vi "Get Area Temperature.vi"(8 "error in (no error)":errorcluster, 10 "Cluster":T1, 11 "Thermal Camera in":refnum<class "Thermal Camera.lvclass">) -> (0 "error out":errorcluster, 1 "Avg Temp":dbl, 2 "Area Temps":dbl[][](array[numeric]), 3 "Thermal Camera out":refnum<class "Thermal Camera.lvclass">)   [LabVIEW 2018, in "Thermal Camera.lvlib" / "Thermal Camera.lvclass"]
uses:
  Thermal Camera.lvclass
  Accessors/Area Coordinates.ctl
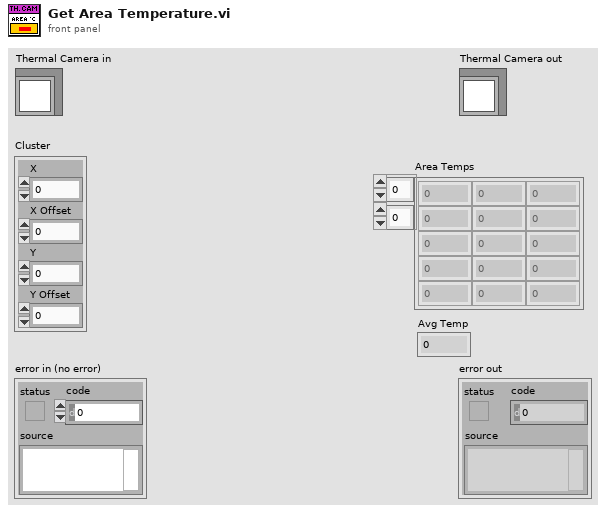
[diagram p1: front panel]
types:
  T1 = typedef "Thermal Camera.lvlib/Thermal Camera.lvclass/Area Coordinates.ctl" = cluster{"X":i32, "X Offset":i32, "Y":i32, "Y Offset":i32}
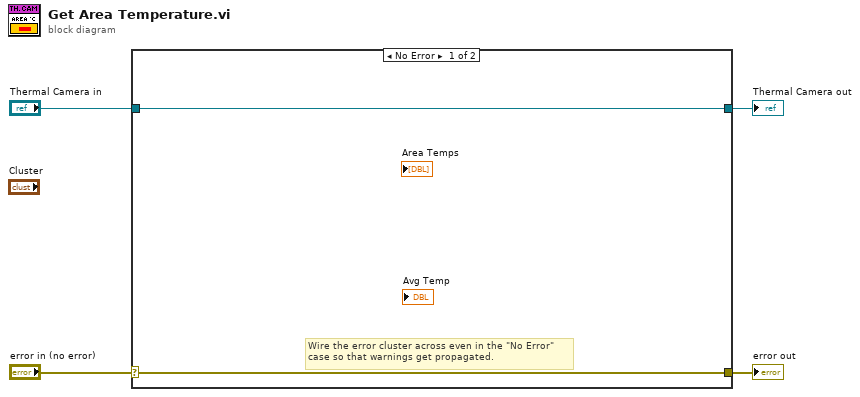
[diagram p0: block diagram]
diagram:
  n1 = case shown="No Error" "error in (no error)" {
    selector: "error in (no error)" -> [w5 w8]
    tunnel: [w5 w8] -> w3
    tunnel: [w6 w7] -> w1
    tunnel: "Thermal Camera in" -> [w6 w7]
    frame No Error {
      # "Wire the error cluster across even in the \"No Error\"\ncase so that warnings get propagated."
    }
    frame Error {
    }
  }
  "error out" <- w3
  "Thermal Camera out" <- w1
